vi "control output Simulation.vi"(10 "DACB":dbl step=0.1 format="%.4f", 11 "DACA":dbl step=0.1 format="%.4f") -> ()   [LabVIEW 2015]
panel:
  out "Torque in-lb":dbl
  in  "stop":bool
  out "Torque output":dbl[](array[numeric])
  in  "FirstFound":bool=TRUE
  in  "Address":string="1"
  out "Error Message":string
  out "error out":errorcluster
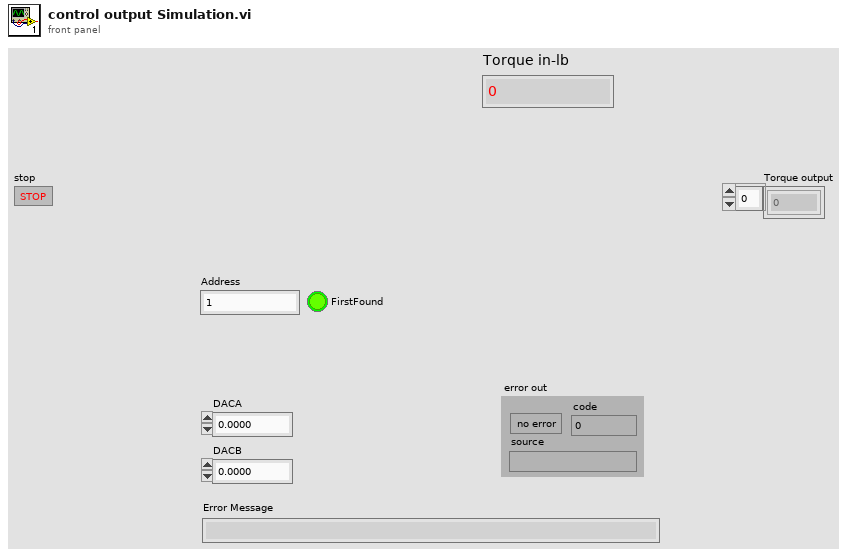
[diagram p1: front panel]
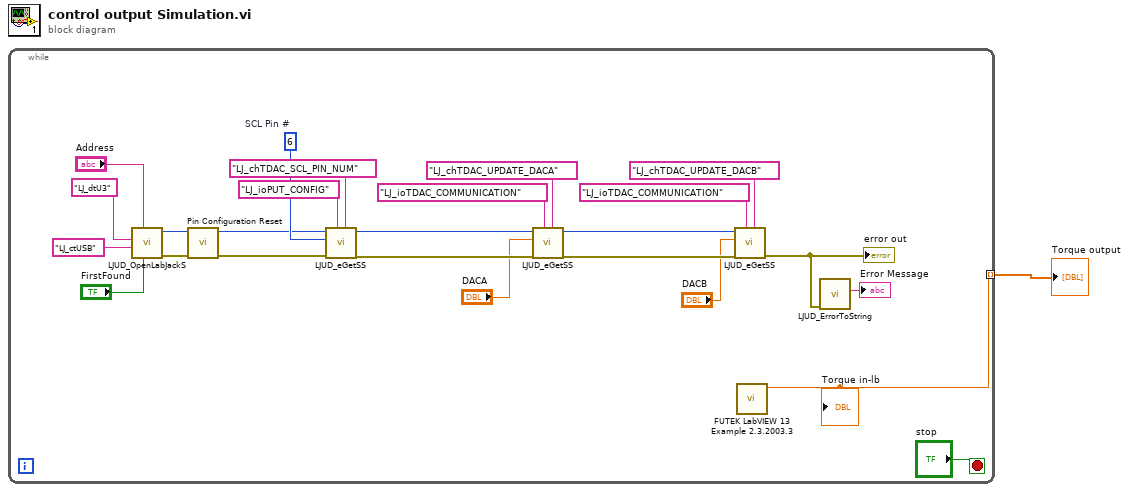
[diagram p0: block diagram]
diagram:
  n1 = while {
    tunnel: [w3] -> w1 mode=indexing
    stop <- "stop" stop-if-true
    w17 = 6  # SCL Pin #
    n2 = call "LJUD_OpenLabJackS.vi"("FirstFound"="FirstFound", "Address"="Address", "ConnectionType"="LJ_ctUSB", "DeviceType"="LJ_dtU3") -> ("error out"=w20:errorcluster, "Handle"=w21:i32)  [unwired: 5 in, 1 out]
    n3 = call "Pin Configuration Reset.vi"("error in"=w20, "Handle In"=w21) -> ("error out"=w15:errorcluster, "Handle Out"=w16:i32)  [unwired: 8 in]
    n4 = call "LJUD_eGetSS.vi"("Channel"="LJ_chTDAC_SCL_PIN_NUM", "IOType"="LJ_ioPUT_CONFIG", "error in"=w15, "Value Write"=w17, "Handle In"=w16) -> ("error out"=w11:errorcluster, "Handle Out"=w12:i32)  [unwired: 4 in, 1 out]
    n5 = call "LJUD_eGetSS.vi"("Channel"="LJ_chTDAC_UPDATE_DACA", "IOType"="LJ_ioTDAC_COMMUNICATION", "error in"=w11, "Value Write"="DACA", "Handle In"=w12) -> ("error out"=w6:errorcluster, "Handle Out"=w7:i32)  [unwired: 4 in, 1 out]
    n6 = call "LJUD_eGetSS.vi"("Channel"="LJ_chTDAC_UPDATE_DACB", "IOType"="LJ_ioTDAC_COMMUNICATION", "error in"=w6, "Value Write"="DACB", "Handle In"=w7) -> ("error out"=w5:errorcluster)  [unwired: 4 in, 2 out]
    "error out" <- w5
    n7 = call "FUTEK LabVIEW 13 Example 2.3.2003.3.vi"() -> ("Torque in-lb"=w3:dbl)  [unwired: 11 in]
    "Torque in-lb" <- w3
    n8 = call "LJUD_ErrorToString.vi"("error in"=w5) -> ("String"=→"Error Message":string)  [unwired: 10 in]
  }
  "Torque output" <- w1
